vi "Save-Recall Waveform.vi"(8 "error in (no error)":errorcluster, 9 "Store Number (1)":dbl(ring)=1.0 items=["1"=1.0, "2"=2.0, "3"=3.0, "4"=4.0], 10 "Waveform Action (Save)":u16(ring) items=["Save", "Recall"], 11 "VISA resource name":refnum<visa-resource-name>) -> (0 "error out":errorcluster, 3 "VISA resource name out":refnum<visa-resource-name>)   [LabVIEW 2015, in "Fluke 28x Series.lvlib"]
doc: "Saves the details of the entire instrument, and recalls those details, in up to 9 memory spaces on the generator."
uses:
  <instrlib>/Fluke 28x Series/Fluke 28x Series.lvlib
panel:
  # "This saves and recalls settings\nfor the entire instrument."
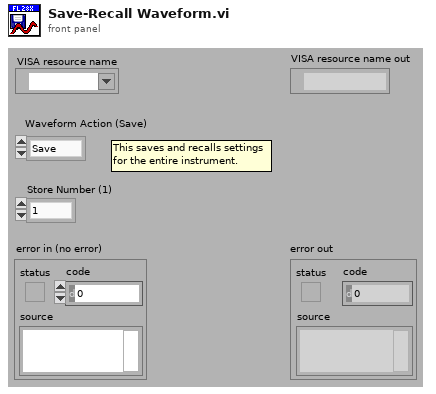
[diagram p1: front panel]
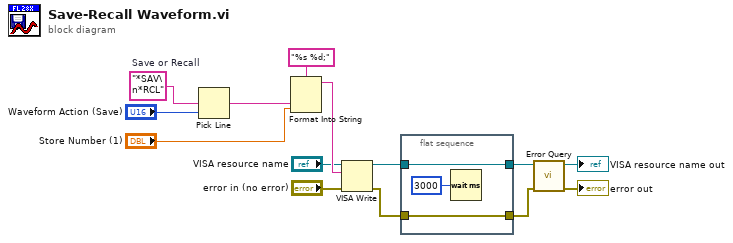
[diagram p0: block diagram]
diagram:
  w14 = "*SAV\n*RCL"  # Save or Recall
  n1 = Pick Line(multi-line string=w14, line index="Waveform Action (Save)") -> (output string=w12:string)  [unwired: 1 in]
  n2 = Format Into String(format string="%s %d;", w12, "Store Number (1)") -> (resulting string=w11:string)  [unwired: 2 in, 1 out]
  n3 = VISA Write(VISA resource name="VISA resource name", write buffer=w11, error in (no error)="error in (no error)") -> (VISA resource name out=w7:refnum<visa-resource-name>, error out=w4:errorcluster)  [unwired: 1 out]
  n4 = flat-sequence {
    tunnel: [w16] -> w6
    tunnel: w7 -> [w16]
    tunnel: [w15] -> w5
    tunnel: w4 -> [w15]
    frame #0 {
      n5 = Wait (ms)(milliseconds to wait=u32 3000) -> ()  [unwired: 1 out]
    }
  }
  n6 = call <instrlib>:"Error Query.vi"("error in (no error)"=w5, "VISA resource name"=w6) -> ("error out"=→"error out":errorcluster, "VISA resource name out"=→"VISA resource name out":refnum<visa-resource-name>)  [unwired: 6 in, 2 out]
